vi "Set Binning.vi"(8 "error in (no error)":errorcluster, 10 "Binning":cluster{"Horizontal":u16, "Vertical":u16}, 11 "Simulated Camera in":refnum<class "Simulated Camera.lvclass">) -> (0 "error out":errorcluster, 2 "Binning out":cluster{"Horizontal":u16, "Vertical":u16}, 3 "Simulated Camera out":refnum<class "Simulated Camera.lvclass">)   [LabVIEW 2019, in "Simulated Camera.lvclass"]
uses:
  Simulated Camera.lvclass
  Simulated Camera.lvclass/Simulated Camera.ctl
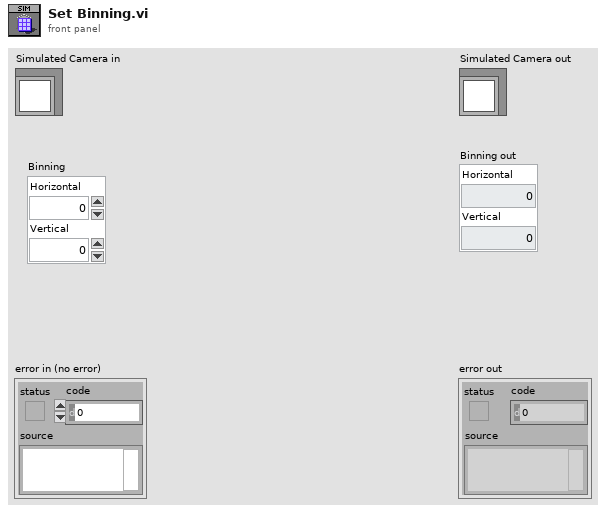
[diagram p1: front panel]
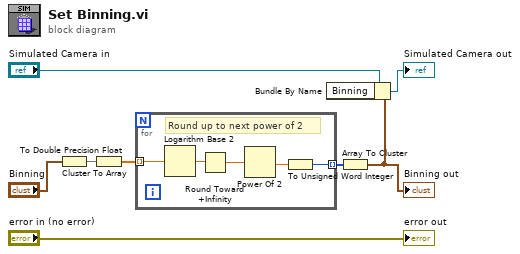
[diagram p0: block diagram]
diagram:
  n1 = Cluster To Array(cluster="Binning") -> (array=w2:u16[])
  n2 = To Double Precision Float(number=w2) -> (double precision float=w7:dbl[])
  n3 = for {
    tunnel: w7 -> [w11] mode=indexing
    tunnel: [w9] -> w8 mode=indexing
    # "Round up to next power of 2"
    n4 = Logarithm Base 2(1:w11) -> (0:w13:dbl)
    n5 = Round Toward +Infinity(x=w13) -> (ceil(x): smallest int >= x=w12:dbl)
    n6 = Power Of 2(x=w12) -> (2^x=w10:dbl)
    n7 = To Unsigned Word Integer(number=w10) -> (unsigned 16bit integer=w9:u16)
  }
  n8 = Array To Cluster(array=w8) -> (cluster=w4:cluster{"[0]":u16, "[1]":u16})
  "Binning out" <- w4
  n9 = Bundle By Name(cluster="Simulated Camera in", "Binning"=w4) -> (→"Simulated Camera out":refnum<class "Simulated Camera.lvclass">)
  "error out" <- "error in (no error)"
